vi "BasicSwitchExecutive Connect.vi"(6 "contextId":T1, 8 "error in":errorcluster, 9 "timeout (ms)":i32=-1, 10 "Request Data":T3, 11 "gRPC ID":T1) -> (0 "error out":errorcluster, 2 "Response Data":T2, 3 "gRPC ID out":T1)   [LabVIEW 2021, in "basic_switch_executive_driver_client.lvlib"]
uses:
  basic_switch_executive_driver_client.lvlib
  <vilib>/gRPC/LabVIEW gRPC Library/Shared/grpcId.ctl
  RPC Messages/nise_ConnectInfo.ctl
  RPC Messages/nise_SessionInformation.ctl
  <vilib>/Plug-In SDKs/Clients/Session Management V1/Session Reservation/Initialize and Close Session Behavior.ctl
  RPC Messages/nise_MulticonnectMode.ctl
  RPC Messages/nise_StatusInfo.ctl
  RPC Messages/nise_StatusInfo_Flat.ctl
  14035477-4c25-4107-8ed5-d0c4ef420ce5.vi
  RPC Messages/RichToFlatnise_SessionInformation.vi
  <vilib>/gRPC/LabVIEW gRPC Library/Shared/TranslateGrpcError.vi
  <vilib>/gRPC/LabVIEW gRPC Library/Shared/Wait On Occurrence Wrapper.vi
  <vilib>/gRPC/LabVIEW gRPC Library/Shared/Wait On Occurence.vi
  <vilib>/gRPC/LabVIEW gRPC Library/Server API/Server/Get Server DLL Path.vi
  <vilib>/Utility/error.llb/Error Cluster From Error Code.vi
  <vilib>/Utility/config.llb/Open Config Data.vi
  <vilib>/Utility/config.llb/Write Key.vi
  <vilib>/Utility/config.llb/Write Key (Boolean).vi
  <vilib>/Utility/config.llb/Not A Config Data Refnum.vi
  <vilib>/Utility/config.llb/Read Key.vi
  <vilib>/Utility/config.llb/Read Key (Boolean).vi
  <vilib>/Utility/config.llb/Close Config Data.vi
  <vilib>/gRPC/LabVIEW gRPC Library/grpc-lvsupport-release.lvlib
  <vilib>/Plug-In SDKs/Clients/Session Management V1/Session Reservation/Session Reservation.lvclass
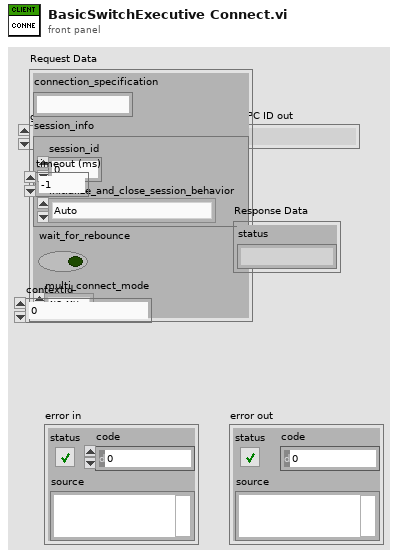
[diagram p1: front panel]
types:
  T1 = typedef "grpc-lvsupport-release.lvlib/grpcId.ctl" = u64
  T2 = typedef "basic_switch_executive_driver_client.lvlib/nise_StatusInfo.ctl" = cluster{"status":string}
  T3 = typedef "basic_switch_executive_driver_client.lvlib/nise_ConnectInfo.ctl" = cluster{"connection_specification":string, "session_info":T4, "wait_for_rebounce":bool, "multi_connect_mode":T6}
  T4 = typedef "basic_switch_executive_driver_client.lvlib/nise_SessionInformation.ctl" = cluster{"session_id":u32, "initialize_and_close_session_behavior":T5}
  T5 = typedef "NI Session Management V1 Client.lvlib/Session Reservation.lvclass/Initialize and Close Session Behavior.ctl" = enum16{"Auto", "Initialize and Close", "Attach and Detach", "Initialize and Detach", "Attach and Close"}
  T6 = typedef "basic_switch_executive_driver_client.lvlib/nise_MulticonnectMode.ctl" = enum32{"NO_MULTICONNECT", "USE_DEFAULT_MODE", "MULTICONNECT_ROUTES"}
  T7 = typedef "basic_switch_executive_driver_client.lvlib/nise_StatusInfo_Flat.ctl" = cluster{"status":string}
  T8 = typedef "basic_switch_executive_driver_client.lvlib/nise_ConnectInfo_Flat.ctl" = cluster{"connection_specification":string, "session_info":T9, "wait_for_rebounce":bool, "multi_connect_mode":T6}
  T9 = typedef "basic_switch_executive_driver_client.lvlib/nise_SessionInformation_Flat.ctl" = cluster{"session_id":u32}
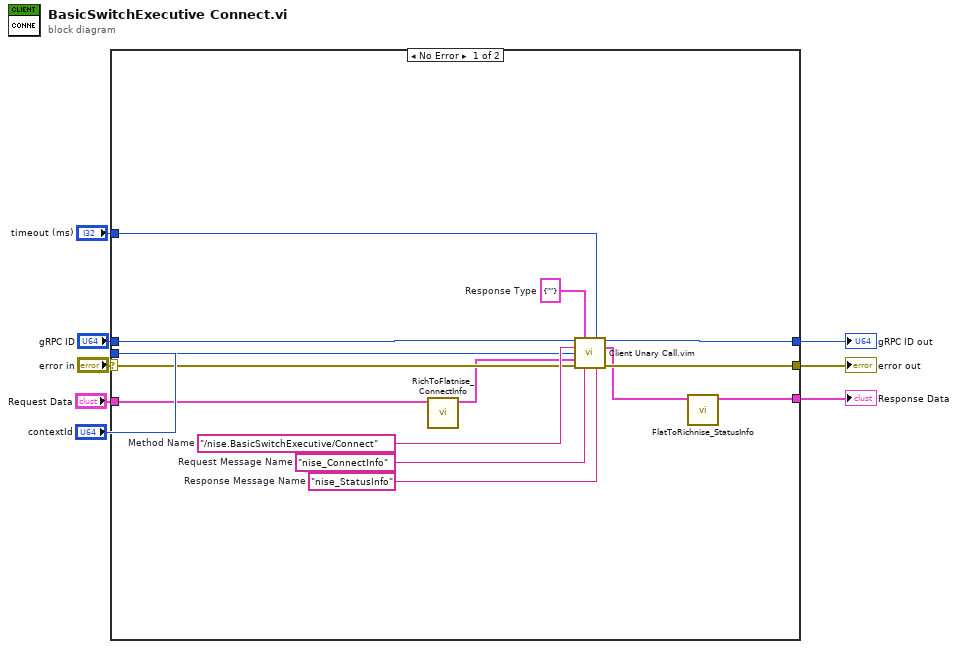
[diagram p0: block diagram]
diagram:
  n1 = case shown="No Error" "error in" {
    selector: "error in" -> [w18 w23]
    tunnel: [w17 w23] -> w7
    tunnel: "gRPC ID" -> [w16 w24]
    tunnel: [w15 w24] -> w5
    tunnel: "Request Data" -> [w12 _]
    tunnel: [w9 _] -> w3
    tunnel: "timeout (ms)" -> [w14 _]
    tunnel: "contextId" -> [w13 _]
    frame No Error {
      w19 = "nise_StatusInfo"  # Response Message Name
      w20 = "nise_ConnectInfo"  # Request Message Name
      w21 = T7 {"status"=""}  # Response Type
      w22 = "/nise.BasicSwitchExecutive/Connect"  # Method Name
      n2 = call "RichToFlatnise_ConnectInfo.vi"("InputCluster"=w12) -> ("OutputCluster"=w11:T8)  [unwired: 10 in]
      n3 = call "Client Unary Call.vim"("ClientID in"=w16, "Response Type"=w21, "timeout (ms)"=w14, "Method Name"=w22, "contextId"=w13, "Request Data"=w11, "error in"=w18, "Request Message Name"=w20, "Response Message Name"=w19) -> ("ClientID out"=w15:u64, "Response Data"=w10:T7, "error out"=w17:errorcluster)  [unwired: 4 in]
      n4 = call "FlatToRichnise_StatusInfo.vi"("InputCluster"=w10) -> ("OutputCluster"=w9:T2)  [unwired: 10 in]
    }
    frame Error {
    }
  }
  "error out" <- w7
  "gRPC ID out" <- w5
  "Response Data" <- w3
